vi "RunM100CRHSocketContactNew.vi"() -> ()   [LabVIEW 2012]
uses:
  <vilib>/addons/database/Connection.llb/DB Tools Open Connec (Path).vi
  <vilib>/addons/database/Connection.llb/Conn Execute.vi
  <vilib>/addons/database/Recordset.llb/Rec Destroy - Connection.vi
  <vilib>/addons/database/NI_Database_API.lvlib
panel:
  out "error out 3":errorcluster
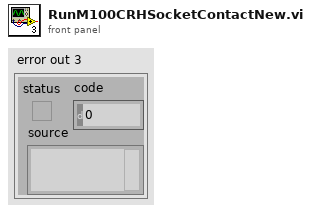
[diagram p1: front panel]
types:
  T1 = typedef "NI_Database_API.lvlib/Conn ObjectReference.ctl" = refnum<k1>
  T2 = typedef "NI_Database_API.lvlib/Rec ObjectReference.ctl" = refnum<k1>
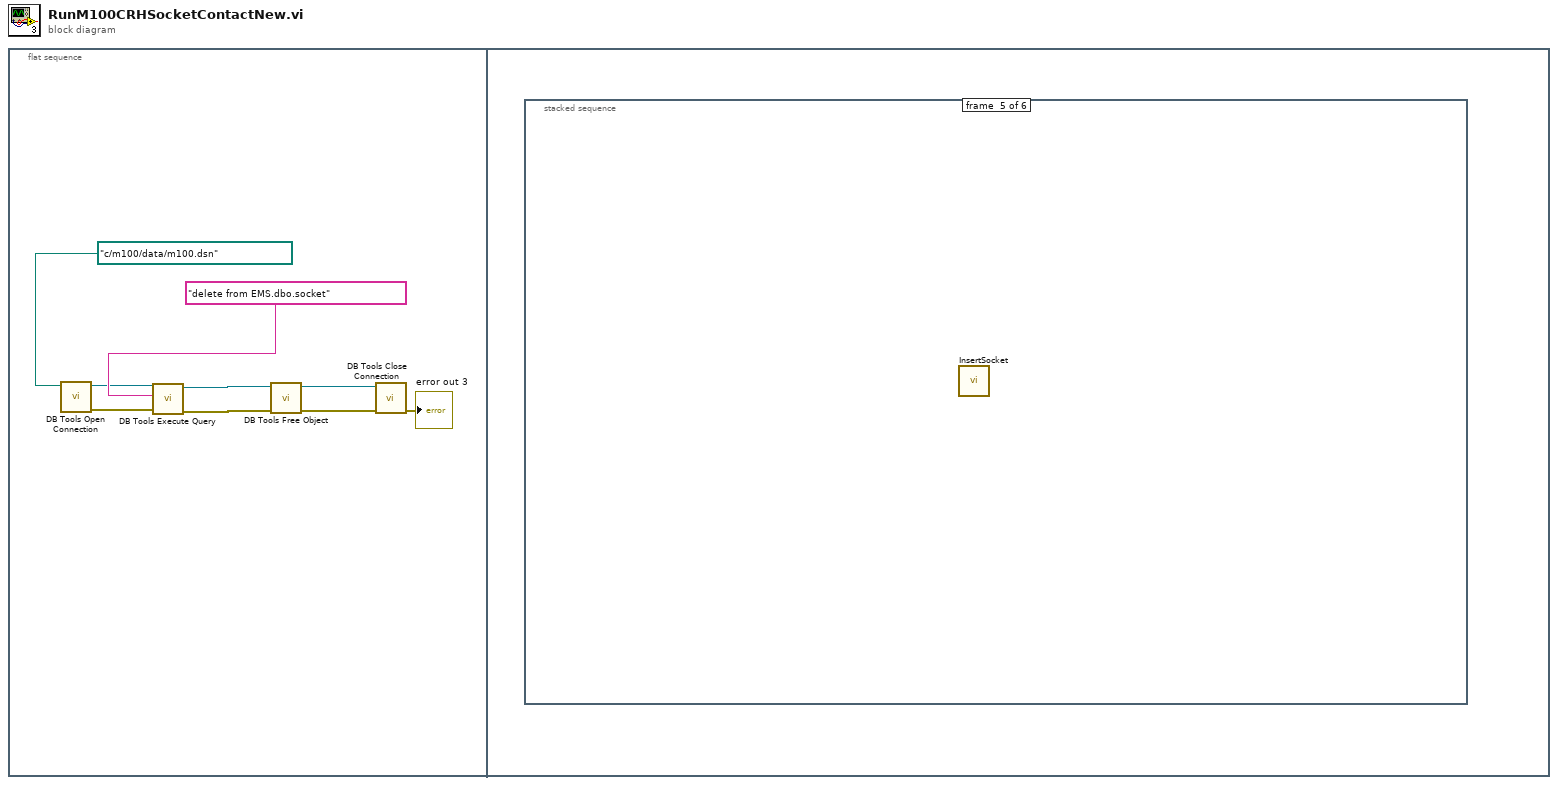
[diagram p0: block diagram]
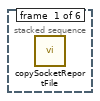
[diagram p2: hidden frame]
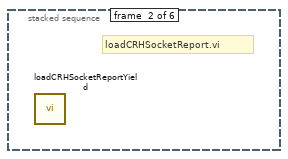
[diagram p3: hidden frame]
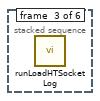
[diagram p4: hidden frame]
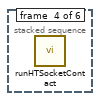
[diagram p5: hidden frame]
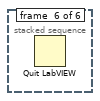
[diagram p6: hidden frame]
diagram:
  n1 = flat-sequence {
    frame #0 {
      n2 = call-poly <vilib>:"DB Tools Open Connection.vi"("connection information"=path "c:/m100/data/m100.dsn") -> ("error out"=w7:errorcluster, "connection reference"=w8:T1)  [unwired: 7 in]
      n3 = call-poly <vilib>:"DB Tools Execute Query.vi"("error in (no error)"=w7, "SQL query"="delete from EMS.dbo.socket", "connection reference"=w8) -> ("error out"=w3:errorcluster, "recordset reference"=w1:T2)  [unwired: 5 in]
      n4 = call-poly <vilib>:"DB Tools Free Object.vi"("error in (no error)"=w3, "recordset reference"=w1) -> ("error out"=w4:errorcluster, "connection reference"=w2:T1)  [unwired: 8 in]
      n5 = call <vilib>:"DB Tools Close Connection.vi"("error in (no error)"=w4, "connection reference"=w2) -> ("error out"=→"error out 3":errorcluster)  [unwired: 5 in]
    }
    frame #1 {
      n6 = stacked-sequence {
        frame #0 {
          n7 = call "copySocketReportFile.vi"() -> ()  [unwired: 12 in]
        }
        frame #1 {
          # "loadCRHSocketReport.vi"
          n8 = call "loadCRHSocketReportYield.vi"() -> ()  [unwired: 12 in]
        }
        frame #2 {
          n9 = call "runLoadHTSocketLog.vi"() -> ()  [unwired: 12 in]
        }
        frame #3 {
          n10 = call "runHTSocketContact.vi"() -> ()  [unwired: 12 in]
        }
        frame #4 {
          n11 = call "InsertSocket.vi"() -> ()  [unwired: 12 in]
        }
        frame #5 {
          n12 = Quit LabVIEW() -> ()  [unwired: 1 in]
        }
      }
    }
  }
